vi "onDestroy.vi"(8 "error in (no error)":errorcluster, 11 "Server in":refnum<class "Server.lvclass">) -> (0 "error out":errorcluster, 3 "Server out":refnum<class "Server.lvclass">)   [LabVIEW 2013, in "MQTT Server.lvlib" / "Server.lvclass"]
uses:
  Server.lvclass
  MQTT_Base/Base Class/MQTT_Base.lvclass
  Server.lvclass/Server.ctl
  StoredSessions/StoredSessions.lvclass
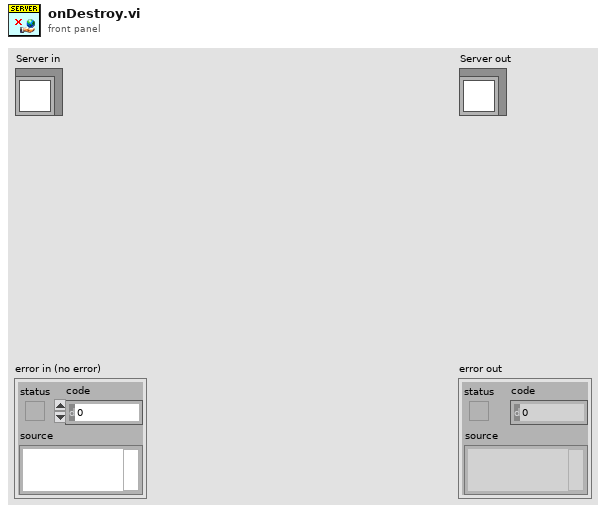
[diagram p1: front panel]
types:
  T1 = typedef "MQTT Server.lvlib/Server.lvclass/SessionRef -- cluster.ctl" = cluster{"ClientID":string, "SessionMailbox":refnum<queue>}
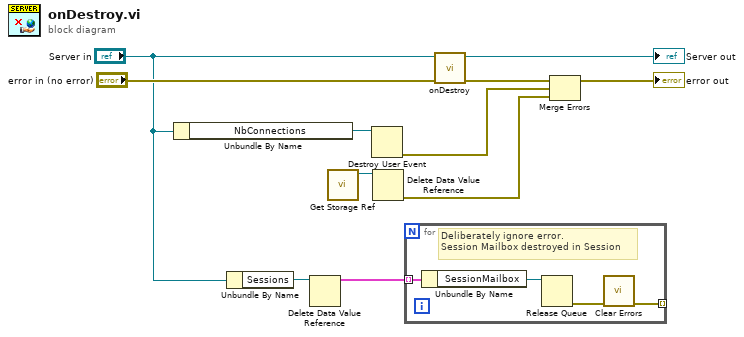
[diagram p0: block diagram]
diagram:
  n1 = Unbundle By Name("Server in") -> ("NbConnections"=w8:refnum<user-event>)
  n2 = Unbundle By Name("Server in") -> ("Sessions"=w1:refnum<data-value>)
  n3 = Delete Data Value Reference(data value reference=w1) -> (data value=w3:T1[])  [unwired: 1 in, 1 out]
  n4 = call "Get Storage Ref.vi"() -> ("Storage"=w10:refnum<data-value>)  [unwired: 11 in]
  n5 = Destroy User Event(user event=w8) -> (error out=w4:errorcluster)  [unwired: 1 in]
  n6 = Delete Data Value Reference(data value reference=w10) -> (error out=w9:errorcluster)  [unwired: 1 in, 1 out]
  n7 = for {
    tunnel: w3 -> [w15] mode=indexing
    tunnel: [w12] -> _ mode=indexing
    # "Deliberately ignore error.\nSession Mailbox destroyed in Session"
    n8 = Unbundle By Name(w15) -> ("SessionMailbox"=w14:refnum<queue>)
    n9 = Release Queue(queue=w14) -> (error out=w13:errorcluster)  [unwired: 2 in, 2 out]
    n10 = call <vilib>:"Clear Errors.vi"("error in (no error)"=w13) -> ("error out"=w12:errorcluster)  [unwired: 6 in]
  }
  n11 = call-parent "onDestroy.vi"("error in (no error)"="error in (no error)", "MQTT_Base in"="Server in") -> ("error out"=w6:errorcluster, "MQTT_Base out"=→"Server out":refnum<class "Server.lvclass">)  [unwired: 8 in]
  n12 = Merge Errors(w6, w4, w9) -> (→"error out":errorcluster)
